vi "Instrument Update Table for Spartan 5.4.vi"(8 "error in (no error)":errorcluster, 11 "Connection Refnum":T1) -> (0 "error out":errorcluster, 3 "Connection Refnum":T1)   [LabVIEW 2011]
uses:
  Summitek EXT/ODBC/SQL Controls/Connection Refnum.ctl
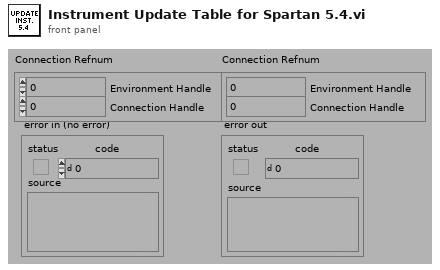
[diagram p1: front panel]
types:
  T1 = typedef "Connection Refnum.ctl" = cluster{"Environment Handle":i32, "Connection Handle":i32}
  T2 = typedef "Statement Refnum.ctl" = cluster{"Statement Handle":i32, "Parameter Number":u16}
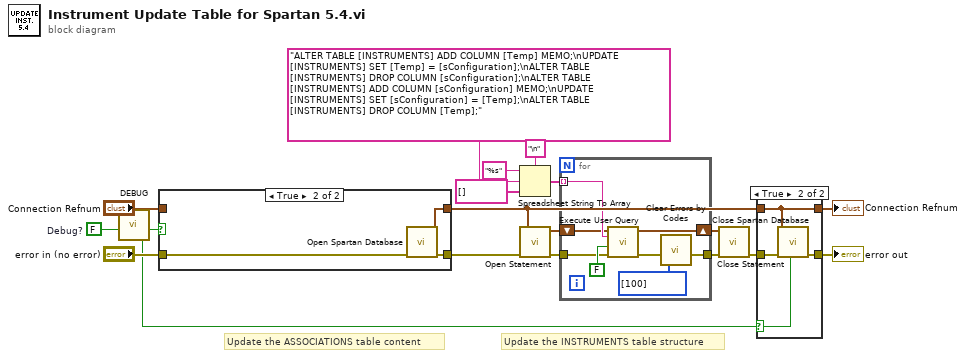
[diagram p0: block diagram]
diagram:
  w6 = FALSE  # Debug?
  # "Update the ASSOCIATIONS table content"
  # "Update the INSTRUMENTS table structure"
  n1 = call "DEBUG.vi"("Dev DEBUG? (f)"=w6) -> ("DEBUG?"=w5:bool)  [unwired: 1 in, 5 out]
  n2 = case shown="True" w5 {
    tunnel: "Connection Refnum" -> [w20 _]
    tunnel: "error in (no error)" -> [w19 w23]
    tunnel: [w19 w22] -> w3
    tunnel: [w20 w21] -> w2
    frame False {
    }
    frame True {
      n3 = call "Open Spartan Database.vi"("error in (no error)"=w23) -> ("error out"=w22:errorcluster, "Connection Refnum"=w21:T1)  [unwired: 2 in, 7 out]
    }
  }
  n4 = Spreadsheet String To Array(delimiter (Tab)="\n", format string="%s", spreadsheet string="ALTER TABLE [INSTRUMENTS] ADD COLUMN [Temp] MEMO;\nUPDATE [INSTRUMENTS] SET [Temp] = [sConfiguration];\nALTER TABLE [INSTRUMENTS] DROP COLUMN [sConfiguration];\nALTER TABLE [INSTRUMENTS] ADD COLUMN [sConfiguration] MEMO;\nUPDATE [INSTRUMENTS] SET [sConfiguration] = [Temp];\nALTER TABLE [INSTRUMENTS] DROP COLUMN [Temp];" ("User Query"), array type (2D Dbl)=string[] []) -> (array=w17:string[])
  n5 = call "Open Statement.vi"("error in (no error)"=w3, "Connection Refnum"=w2) -> ("error out"=w14:errorcluster, "Statement Refnum"=w13:T2)  [unwired: 4 out]
  n6 = for {
    tunnel: w17 -> [w30] mode=indexing
    shift-right: [w27] -> w11
    shift-left: w13 -> [w29]
    tunnel: w14 -> [w28]
    tunnel: [w24] -> w12
    n7 = call "Execute User Query.vi"("error in (no error)"=w28, "Return Data? (f)"=FALSE, "User Query"=w30, "Statement Refnum"=w29) -> ("error out"=w25:errorcluster, "Statement Refnum"=w27:T2)  [unwired: 2 out]
    n8 = call "Clear Errors by Codes.vi"("Error Codes\nto Clear (Empty)"=i32[] [100] ("Error Codes\nto Clear (Empty)"), "error in (no error)"=w25) -> ("error out"=w24:errorcluster)  [unwired: 5 out]
  }
  n9 = call "Close Statement.vi"("error in (no error)"=w12, "Statement Refnum"=w11) -> ("error out"=w1:errorcluster)  [unwired: 5 out]
  n10 = case shown="True" w5 {
    selector: w5 -> [_ w35]
    tunnel: w1 -> [w33 w37]
    tunnel: w2 -> [w32 w34]
    tunnel: [w32 w34] -> w10
    tunnel: [w33 w36] -> w9
    frame False {
    }
    frame True {
      n11 = call "Close Spartan Database.vi"("Force Close? (f)"=w35, "error in (no error)"=w37, "Connection Refnum"=w34) -> ("error out"=w36:errorcluster)  [unwired: 2 in, 6 out]
    }
  }
  "error out" <- w9
  "Connection Refnum" <- w10
